vi "Initialize Hardware.vi"(7 "hardware config file":path, 8 "error in":errorcluster, 10 "number of ports":i32, 11 "device parameters":T2) -> (0 "error out":errorcluster, 3 "module reference":T1)   [LabVIEW 2020, in "AIM MIL-STD-1553 Engine.lvlib" / "Custom Device.lvlib"]
uses:
  Custom Device.lvlib
  <instrlib>/BTICardLib/BTICardLV.lvlib
  <instrlib>/BTICardLib/Private/IO/Action-Status/Write External LED.vi
  <instrlib>/BTI1553Lib/BTI1553LV.lvlib
  Hardware Handles.ctl
  <instrlib>/BTICardLib/Private/Initialize By Card Number and Core Number.vi
  <instrlib>/BTICardLib/Private/Initialize By Slot Number and Core Number.vi
  <instrlib>/BTI1553Lib/Private/Channel/Configure/Configure All From XML.vi
  Wrapped AIM Palette/AIM MIL-STD-1553 Wrapped Palette.lvlib
  Shared/Device Parameters.ctl
  Shared/Initialization Method.ctl
  Wrapped AIM Palette/Module Reference.ctl
panel:
  out "type string out":string
  out "product string out":string
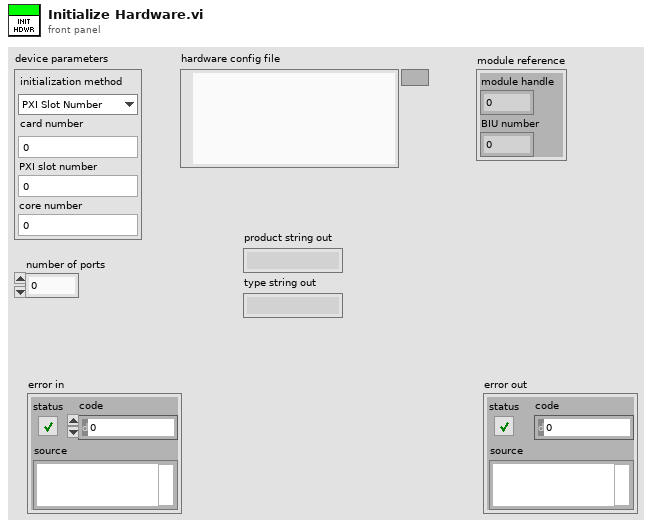
[diagram p1: front panel]
types:
  T1 = typedef "AIM MIL-STD-1553 Wrapped Palette.lvlib/Module Reference.ctl" = cluster{"module handle":u32, "BIU number":u8}
  T2 = typedef "Device Parameters.ctl" = cluster{"initialization method":T3, "card number":i32, "PXI slot number":i32, "core number":i32}
  T3 = typedef "Initialization Method.ctl" = enum16{"PXI Slot Number", "Card Number"}
  T4 = typedef "AIM MIL-STD-1553 Engine.lvlib/Custom Device.lvlib/Hardware Handles.ctl" = cluster{"core handle":u64, "core reader handle":u64, "channel handles":u64[]}
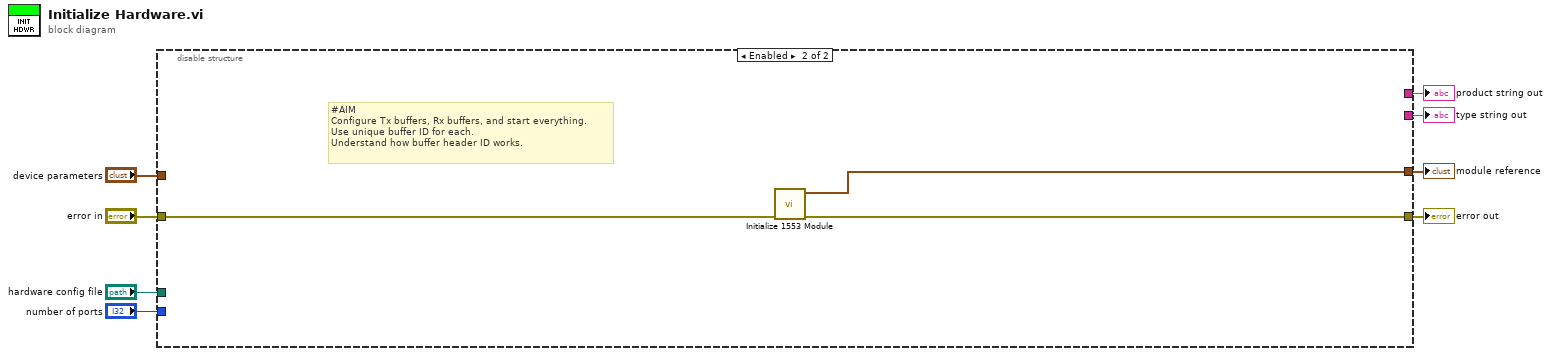
[diagram p0: block diagram]
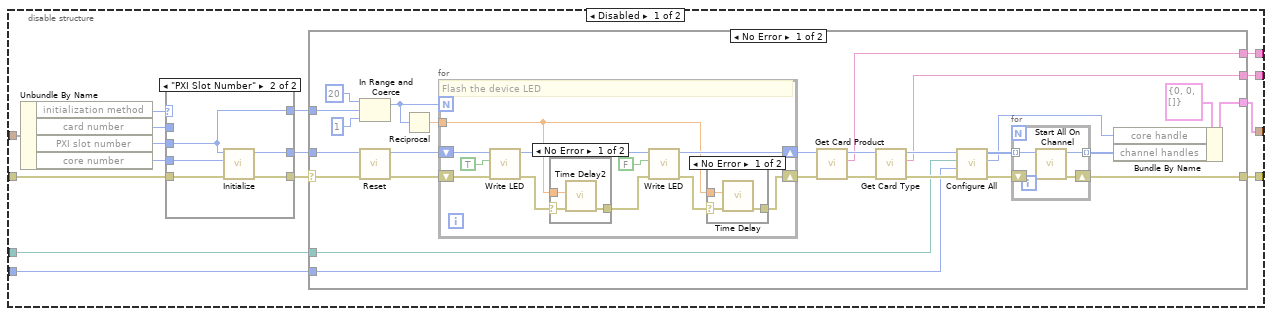
[diagram p2: hidden frame]
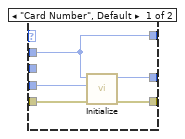
[diagram p3: hidden frame]
diagram:
  n1 = disable-structure shown="Enabled" {
    disable-tunnel: "device parameters" -> [w23 _]
    disable-tunnel: "hardware config file" -> [w22 _]
    disable-tunnel: [w21 w86] -> w6
    disable-tunnel: [w20 w84] -> w1
    disable-tunnel: "error in" -> [w13 w85]
    disable-tunnel: "number of ports" -> [w11 _]
    disable-tunnel: [w10 _] -> w3
    disable-tunnel: [w9 _] -> w2
    frame Disabled {
      n2 = Unbundle By Name(w23) -> ("initialization method"=w16:T3, "card number"=w15:i32, "PXI slot number"=w19:i32, "core number"=w17:i32)
      n3 = case shown="\"PXI Slot Number\"" w16 {
        tunnel: [w28 w33] -> w14
        tunnel: [w27 w32] -> w12
        tunnel: w15 -> [w24 _]
        tunnel: w13 -> [w26 w31]
        tunnel: w19 -> [_ w29]
        tunnel: w17 -> [w25 w30]
        tunnel: [w24 w29] -> w18
        frame "Card Number", Default {
          n4 = call-poly <instrlib>:"Initialize.vi"("error in (no error)"=w26, "core number"=w25, "card number"=w24) -> ("error out"=w27:errorcluster, "core handle out"=w28:u64)  [unwired: 7 in]
        }
        frame "PXI Slot Number" {
          n5 = call-poly <instrlib>:"Initialize.vi"("error in (no error)"=w31, "core number"=w30, "slot number"=w29) -> ("error out"=w32:errorcluster, "core handle out"=w33:u64)  [unwired: 7 in]
        }
      }
      n6 = case shown="No Error" w12 {
        selector: w12 -> [w52 w83]
        tunnel: w14 -> [w53 _]
        tunnel: w18 -> [w51 _]
        tunnel: w22 -> [w44 _]
        tunnel: [w41 w83] -> w21
        tunnel: [w34 _] -> w20
        tunnel: w11 -> [w38 _]
        tunnel: [w37 _] -> w10
        tunnel: [w36 _] -> w9
        frame No Error {
          n7 = In Range and Coerce(upper limit=20 ("x"), x=w51, lower limit=1) -> (coerced(x)=w59:i32)  [unwired: 1 out]
          n8 = call <instrlib>:"Reset.vi"("error in (no error)"=w52, "core handle in"=w53) -> ("error out"=w54:errorcluster, "core handle out"=w55:u64)  [unwired: 8 in]
          n9 = Reciprocal(x=w59) -> (1/x=w58:dbl)
          n10 = for {
            N: w59 -> [_]
            shift-right: [w73] -> w46
            shift-left: w55 -> [w72]
            shift-right: [w67] -> w45
            shift-left: w54 -> [w71]
            tunnel: w58 -> [w64]
            # "Flash the device LED"
            n11 = call-poly <instrlib>:"Write LED.vi"("error in (no error)"=w71, "LED state"=TRUE, "core handle in"=w72) -> ("error out"=w66:errorcluster, "core handle out"=w74:u64)  [unwired: 7 in]
            n12 = case shown="No Error" w66 {
              selector: w66 -> [w77 w78]
              tunnel: [w76 w78] -> w65
              tunnel: w64 -> [w75 _]
              frame No Error {
                n13 = call "Time Delay2"("error in (no error)"=w77, "Delay Time (s)"=w75) -> ("error out"=w76:errorcluster)  [unwired: 9 in]
              }
              frame Error {
              }
            }
            n14 = call-poly <instrlib>:"Write LED.vi"("error in (no error)"=w65, "LED state"=FALSE, "core handle in"=w74) -> ("error out"=w68:errorcluster, "core handle out"=w73:u64)  [unwired: 7 in]
            n15 = case shown="No Error" w68 {
              selector: w68 -> [w81 w82]
              tunnel: [w80 w82] -> w67
              tunnel: w64 -> [w79 _]
              frame No Error {
                n16 = call "Time Delay"("error in (no error)"=w81, "Delay Time (s)"=w79) -> ("error out"=w80:errorcluster)  [unwired: 9 in]
              }
              frame Error {
              }
            }
          }
          n17 = call <instrlib>:"Get Card Product.vi"("error in (no error)"=w45, "core handle in"=w46) -> ("error out"=w48:errorcluster, "product string out"=w36:string, "core handle out"=w47:u64)  [unwired: 7 in]
          n18 = call <instrlib>:"Get Card Type.vi"("error in (no error)"=w48, "core handle in"=w47) -> ("error out"=w50:errorcluster, "type string out"=w37:string, "core handle out"=w49:u64)  [unwired: 7 in]
          n19 = call-poly <instrlib>:"Configure All.vi"("error in (no error)"=w50, "channel handle array size in"=w38, "configuration file path"=w44, "core handle in"=w49) -> ("error out"=w42:errorcluster, "core handle out"=w35:u64, "channel handles out"=w43:u64[])  [unwired: 4 in, 1 out]
          n20 = for {
            tunnel: w43 -> [w63] mode=indexing
            tunnel: [w60] -> w39 mode=indexing
            shift-right: [w61] -> w41
            shift-left: w42 -> [w62]
            n21 = call <instrlib>:"Start All On Channel.vi"("error in (no error)"=w62, "channel handle in"=w63) -> ("error out"=w61:errorcluster, "channel handle out"=w60:u64)  [unwired: 8 in]
          }
          n22 = Bundle By Name(cluster=T4 {"core handle"=0, "core reader handle"=0, "channel handles"=[]} ("hardware handles"), "core handle"=w35, "channel handles"=w39) -> (w34:T4)
        }
        frame Error {
        }
      }
    }
    frame Enabled {
      # "#AIM\nConfigure Tx buffers, Rx buffers, and start everything.\nUse unique buffer ID for each.\nUnderstand how buffer header ID works."
      n23 = call "Initialize 1553 Module.vi"("error in"=w85) -> ("error out"=w86:errorcluster, "module reference"=w84:T1)  [unwired: 9 in]
    }
  }
  "error out" <- w6
  "type string out" <- w3
  "product string out" <- w2
  "module reference" <- w1
